vi "Configure Connection Dialog.vi"(8 "error in (no error)":errorcluster, 10 "Current Connection":T6, 11 "Channel Editor State":T4={"Controller"="", "Possible Connections"=[{"Module"="", "Possible Connections"=[]}, {"Module"="", "Possible Connections"=[]}], "Alias Mappings UI"=[], "Mappings by Module UI"=[]}) -> (0 "error out":errorcluster, 1 "Connection (R,S,D)":T5, 2 "Canceled?":bool)   [LabVIEW 2017, in "Routing and Faulting System Explorer.lvlib"]
uses:
  Routing and Faulting System Explorer.lvlib
  Connection Row.ctl
  Shared/Connection.ctl
  Shared/Routing and Faulting Hardware API/Types/Possible Connections for Endpoint.ctl
  Shared/Alias Mapping.ctl
  Alias Map by Module.ctl
  <vilib>/event_ctls.llb/lveventtype.ctl
  Shared/Routing and Faulting Shared.lvlib
  Shared/Routing and Faulting Hardware API/Routing and Faulting Hardware API.lvlib
panel:
  out "Module Index":i32
  out "Initial Module":string
  out "Initial Destination":string
  out "Initial Source":string
  in  "Module":string(combo)
  in  "Cancel Button":bool
  in  "OK Button":bool
  in  "Destination":string(combo)
  in  "Source":string(combo)
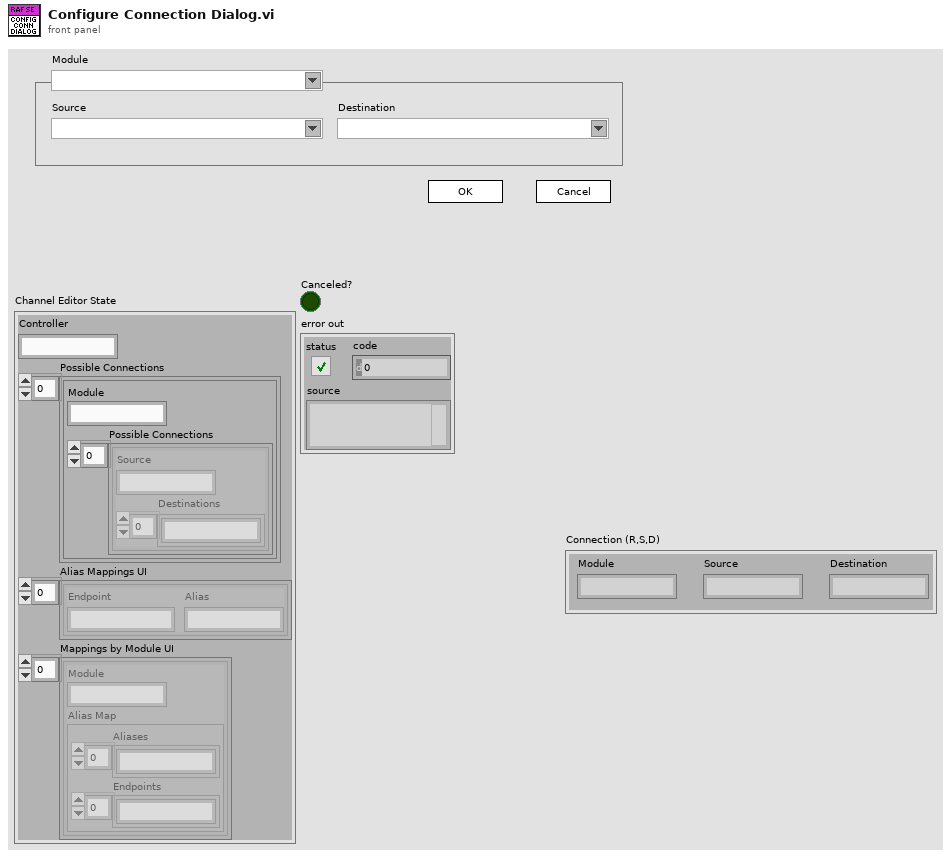
[diagram p1: front panel]
types:
  T1 = typedef "Routing and Faulting Hardware API.lvlib/Possible Connections for Endpoint.ctl" = cluster{"Source":string, "Destinations":string[]}
  T2 = typedef "Routing and Faulting Shared.lvlib/Alias Mapping.ctl" = cluster{"Endpoint":string, "Alias":string}
  T3 = typedef "Routing and Faulting System Explorer.lvlib/Alias Map by Module.ctl" = cluster{"Module":string, "Alias Map":cluster{"Aliases":string[], "Endpoints":string[]}}
  T4 = cluster{"Controller":string, "Possible Connections":cluster{"Module":string, "Possible Connections":T1[]}[], "Alias Mappings UI":T2[], "Mappings by Module UI":T3[]}
  T5 = typedef "Routing and Faulting Shared.lvlib/Connection.ctl" = cluster{"Module":string, "Source":string, "Destination":string}
  T6 = typedef "Routing and Faulting System Explorer.lvlib/Connection Row.ctl" = cluster{"Source":string, "Destination":string, "Edit":bool, "Remove":bool}
  T7 = cluster{"Module":string, "Possible Connections":T1[]}[]
  T8 = typedef "lveventtype.ctl" = enum32{"Null", "Timeout", "Annotation Menu Selection", "Annotation Menu Selection?", "App Instance Close", "App Instance Close?", "Autoscale Range Change", "Bookmark Info Change", "Cell Edit", "Cell Edit?", "Cursor Grab", "Cursor Grab?", "Cursor Menu Selection", "Cursor Menu Selection?", "Cursor Move", "Cursor Release", "Data Change", "Direction Change", "Display State Change", "Drag Ended", "Drag Enter", "Drag Leave", "Drag Over", "Drag Source Update", "Drag Starting", "Drag Starting?", "Drop", "Exec State Change", "Key Down", "Key Down?", "Key Repeat", "Key Repeat?", "Key Up", "Listbox Double Click", "Menu Activation?", "Menu Selection (App)", "Menu Selection? (App)", "Menu Selection (User)", "Mouse Down", "Mouse Down?", "Mouse Enter", "Mouse Leave", "Mouse Move", "Mouse Up", "Mouse Wheel", "NI Security User Change (App)", "Pane Size", "Panel Close", "Panel Close?", "Panel Resize", "Plot Attribute Change", "Scale Range Change", "Shortcut Menu Activation?", "Shortcut Menu Selection (App)", "Shortcut Menu Selection? (App)", "Shortcut Menu Selection (User)", "Tree Double Click", "Tree Drag", "Tree Drag?", "Tree Drop", "Tree Drop?", "Tree Item Close", "Tree Item Close?", "Tree Item Open", "Tree Item Open?", "User Event", "Value Change"}
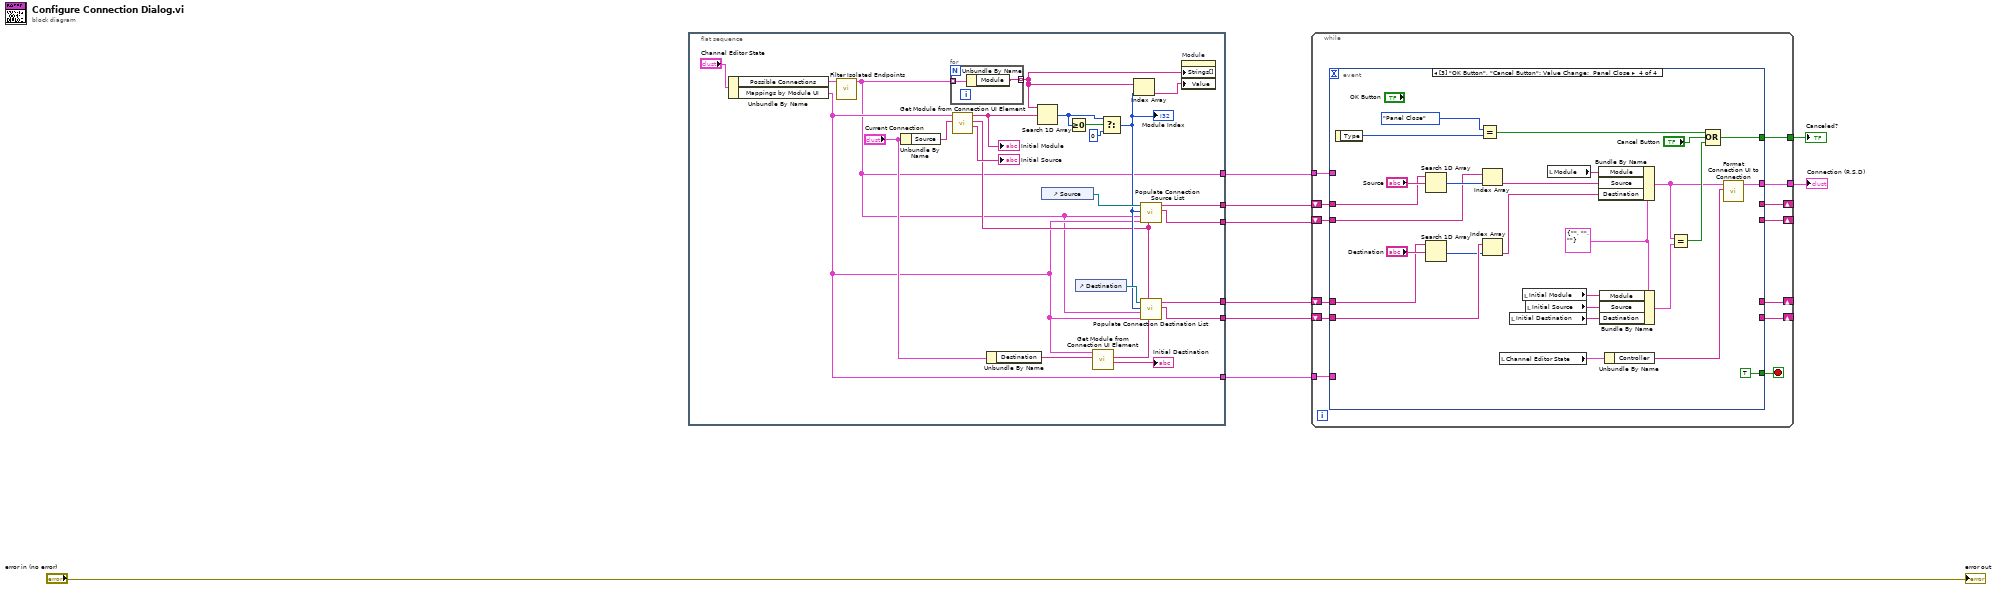
[diagram p0: block diagram]
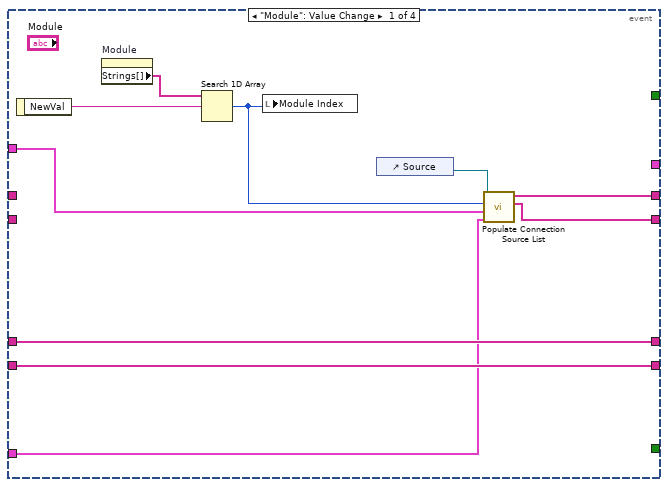
[diagram p2: hidden frame]
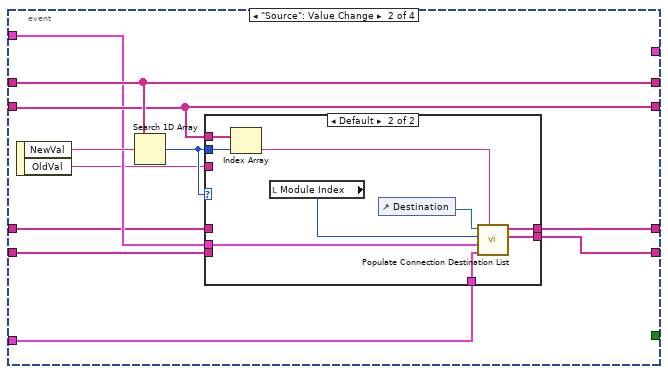
[diagram p3: hidden frame]
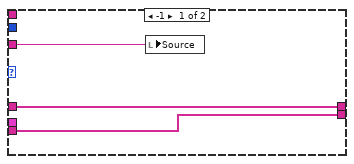
[diagram p4: hidden frame]
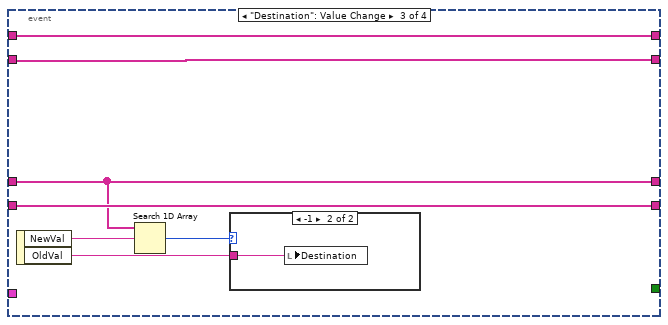
[diagram p5: hidden frame]
diagram:
  n1 = flat-sequence {
    tunnel: [w29] -> w6
    tunnel: [w12] -> w1
    tunnel: [w26] -> w5
    tunnel: [w25] -> w4
    tunnel: [w10] -> w3
    tunnel: [w28] -> w2
    frame #0 {
      n2 = Unbundle By Name("Channel Editor State") -> ("Possible Connections"=w11:T7, "Mappings by Module UI"=w12:T3[])
      n3 = call "Filter Isolated Endpoints.vi"("Possible Connections in"=w11) -> ("Possible Connections out"=w10:T7)  [unwired: 10 in]
      n4 = Unbundle By Name("Current Connection") -> ("Source"=w19:string)
      n5 = for {
        tunnel: w10 -> [w35] mode=indexing
        tunnel: [w34] -> w33 mode=indexing
        n6 = Unbundle By Name(w35) -> ("Module"=w34:string)
      }
      n7 = call "Get Module from Connection UI Element.vi"("Alias or Full Endpoint"=w19, "Alias Mappings by Module"=w12) -> ("Long Endpoint"=→"Initial Source":string, "Short Endpoint"=w17:string, "Module"=w31:string)  [unwired: 7 in]
      "Initial Module" <- w31
      n8 = Unbundle By Name("Current Connection") -> ("Destination"=w16:string)
      n9 = Search 1D Array(1D array=w33, element=w31) -> (index of element=w23:i32)  [unwired: 1 in]
      n10 = control-ref of="Source"() -> (w30:refnum<vi>)
      n11 = Greater Or Equal To 0?(x=w23) -> (x >= 0?=w24:bool)
      n12 = control-ref of="Destination"() -> (w27:refnum<vi>)
      n13 = call "Get Module from Connection UI Element.vi"("Alias or Full Endpoint"=w16, "Alias Mappings by Module"=w12) -> ("Long Endpoint"=→"Initial Destination":string, "Short Endpoint"=w14:string)  [unwired: 7 in, 1 out]
      n14 = Select(t=w23, s=w24, f=0) -> (s? t:f=w20:i32)
      "Module Index" <- w20
      n15 = Index Array(array=w33, index=w20) -> (element=w32:string)
      n16 = call "Populate Connection Source List.vi"("initial Source"=w17, "Alias Mappings by Module"=w12, "Possible Connections"=w10, "Module Index"=w20, "Source Reference"=w30) -> ("Endpoint List"=w28:string[], "Alias List"=w29:string[])  [unwired: 5 in]
      n17 = call "Populate Connection Destination List.vi"("initial Destination"=w14, "Source"=w17, "Alias Mappings by Module"=w12, "Possible Connections"=w10, "Module Index"=w20, "Destination Reference"=w27) -> ("Endpoint List"=w25:string[], "Alias List"=w26:string[])  [unwired: 4 in]
      n18 = property on="Module" class="CmbBox"("Strings[]"=w33, "Value"=w32) -> ()  [unwired: 2 in, 2 out]
    }
  }
  n19 = while {
    tunnel: [w47] -> w9
    tunnel: w3 -> [w46]
    tunnel: [w45] -> w7
    shift-right: [w41] -> _
    shift-left: w6 -> [w44]
    shift-right: [w40] -> _
    shift-left: w2 -> [w43]
    tunnel: w1 -> [w42]
    shift-right: [w39] -> _
    shift-left: w5 -> [w37]
    shift-right: [w38] -> _
    shift-left: w4 -> [w36]
    stop <- w48 stop-if-true
    n20 = event shown="[3] \"OK Button\", \"Cancel Button\": Value Change;  Panel Close" {
      selector: _ -> [_ _ _ _]
      dyn-events: _ -> [_ _ _ _]
      timeout: _ -> [_ _ _ _]
      tunnel: [_ _ _ TRUE] -> w48
      tunnel: [_ _ _ w112] -> w47
      tunnel: w46 -> [w51 w64 _ _]
      tunnel: [_ _ _ w92] -> w45
      tunnel: w44 -> [_ w68 w87 w108]
      tunnel: w43 -> [_ w65 w86 w107]
      tunnel: w42 -> [w52 w63 _ _]
      tunnel: [w57 w68 w87 _] -> w41
      tunnel: [w56 w65 w86 _] -> w40
      tunnel: [w55 w67 w84 _] -> w39
      tunnel: [w54 w66 w85 _] -> w38
      tunnel: w37 -> [w55 w61 w84 w104]
      tunnel: w36 -> [w54 w60 w85 w103]
      event "Module": Value Change {
        n21 = event-data() -> ("NewVal"=w58:string)  [unwired: 1 in]
        n22 = property on="Module" class="CmbBox"() -> ("Strings[]"=w50:string[])  [unwired: 2 in, 2 out]
        n23 = Search 1D Array(1D array=w50, element=w58) -> (index of element=w49:i32)  [unwired: 1 in]
        n24 = local write "Module Index"(w49) -> ()
        n25 = control-ref of="Source"() -> (w53:refnum<vi>)
        n26 = call "Populate Connection Source List.vi"("Alias Mappings by Module"=w52, "Possible Connections"=w51, "Module Index"=w49, "Source Reference"=w53) -> ("Endpoint List"=w56:string[], "Alias List"=w57:string[])  [unwired: 6 in]
      }
      event "Source": Value Change {
        n27 = event-data() -> ("NewVal"=w69:string, "OldVal"=w59:string)  [unwired: 1 in]
        n28 = Search 1D Array(1D array=w68, element=w69) -> (index of element=w62:i32)  [unwired: 1 in]
        n29 = case shown="Default" w62 {
          tunnel: w62 -> [_ w81]
          tunnel: [w72 w80] -> w67
          tunnel: [w71 w79] -> w66
          tunnel: w65 -> [_ w78]
          tunnel: w64 -> [_ w76]
          tunnel: w63 -> [_ w74]
          tunnel: w61 -> [w72 _]
          tunnel: w60 -> [w71 _]
          tunnel: w59 -> [w70 _]
          frame -1 {
            n30 = local write "Source"(w70) -> ()
          }
          frame Default {
            n31 = Index Array(array=w78, index=w81) -> (element=w73:string)
            n32 = local read "Module Index"() -> (w77:i32)
            n33 = control-ref of="Destination"() -> (w75:refnum<vi>)
            n34 = call "Populate Connection Destination List.vi"("Source"=w73, "Alias Mappings by Module"=w74, "Possible Connections"=w76, "Module Index"=w77, "Destination Reference"=w75) -> ("Endpoint List"=w79:string[], "Alias List"=w80:string[])  [unwired: 5 in]
          }
        }
      }
      event "Destination": Value Change {
        n35 = event-data() -> ("NewVal"=w88:string, "OldVal"=w82:string)  [unwired: 1 in]
        n36 = Search 1D Array(1D array=w84, element=w88) -> (index of element=w83:i32)  [unwired: 1 in]
        n37 = case shown="-1" w83 {
          tunnel: w82 -> [_ w89]
          frame Default {
          }
          frame -1 {
            n38 = local write "Destination"(w89) -> ()
          }
        }
      }
      event "OK Button", "Cancel Button": Value Change; Panel Close {
        w100 = T5 {"Module"="", "Source"="", "Destination"=""} ("Connection (R,S,D)")
        n39 = event-data() -> ("Type"=w114:T8)  [unwired: 1 in]
        n40 = Search 1D Array(1D array=w108, element="Source") -> (index of element=w110:i32)  [unwired: 1 in]
        n41 = Search 1D Array(1D array=w104, element="Destination") -> (index of element=w102:i32)  [unwired: 1 in]
        n42 = Equal?(x=lveventtype."Panel Close" ("Type"), y=w114) -> (x = y?=w95:bool)
        n43 = Index Array(array=w107, index=w110) -> (element=w106:string)
        n44 = Index Array(array=w103, index=w102) -> (element=w101:string)
        n45 = local read "Channel Editor State"() -> (w91:T4)
        n46 = local read "Initial Destination"() -> (w96:string)
        n47 = local read "Initial Module"() -> (w98:string)
        n48 = local read "Initial Source"() -> (w97:string)
        n49 = local read "Module"() -> (w111:string)
        n50 = Bundle By Name(cluster=w100, "Module"=w111, "Source"=w106, "Destination"=w101) -> (w93:T5)
        n51 = Bundle By Name(cluster=w100, "Module"=w98, "Source"=w97, "Destination"=w96) -> (w99:T5)
        n52 = Unbundle By Name(w91) -> ("Controller"=w90:string)
        n53 = Equal?(x=w93, y=w99) -> (x = y?=w94:bool)
        n54 = Compound Arithmetic op=OR(w95, "Cancel Button", w94) -> (w112:bool)
        n55 = call "Format Connection UI to Connection.vi"("Controller"=w90, "Connection UI"=w93) -> ("Connection"=w92:T5)  [unwired: 9 in]
      }
    }
  }
  "Canceled?" <- w9
  "Connection (R,S,D)" <- w7
  "error out" <- "error in (no error)"
